vi "updateTestParameters.vi"(8 "error in (no error)":errorcluster, 11 "Model in":refnum<class "Model.lvclass">) -> (0 "error out":errorcluster, 3 "Model out":refnum<class "Model.lvclass">)   [LabVIEW 2015]
uses:
  ApplicationElements/TestMonitor/TestMonitor.lvclass
  Configuration/CycleProfileConfig.ctl
  Configuration/TestParameters.ctl
  ConfigurationThisComponent/ConfigurationThisComponent.lvclass
  Model.lvclass
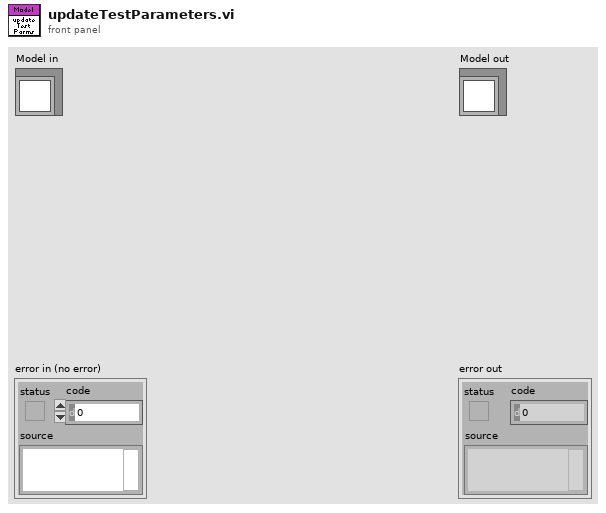
[diagram p1: front panel]
types:
  T1 = typedef "TestParameters.ctl" = cluster{"Number of cycles for complete test":u32, "Cycle profile":T2}
  T2 = typedef "CycleProfileConfig.ctl" = cluster{"Force Setpoint":dbl[unit][], "Pause After":dbl[unit][]}
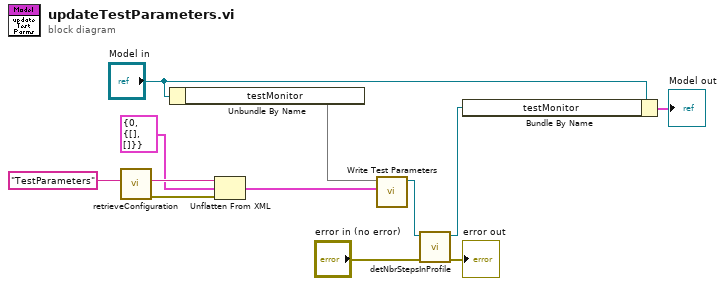
[diagram p0: block diagram]
diagram:
  n1 = call "retrieveConfiguration.vi"("configName"="TestParameters") -> ("error out"=w4:errorcluster, "xmlConfig"=w3:string)  [unwired: 8 in, 1 out]
  n2 = Unbundle By Name("Model in") -> ("testMonitor"=w11)
  n3 = Unflatten From XML(xml string=w3, type=T1 {"Number of cycles for complete test"=0, "Cycle profile"={"Force Setpoint"=[], "Pause After"=[]}} ("Test Parameters"), error in (no error)=w4) -> (value=w1:T1)  [unwired: 1 out]
  n4 = call "Write Test Parameters.vi"("Test Parameters"=w1, "TestMonitor in"=w11) -> ("TestMonitor out"=w10:refnum<class "TestMonitor.lvclass">)  [unwired: 9 in]
  n5 = call "detNbrStepsInProfile.vi"("error in (no error)"="error in (no error)", "TestMonitor in"=w10) -> ("error out"=→"error out":errorcluster, "TestMonitor out"=w9:refnum<class "TestMonitor.lvclass">)  [unwired: 8 in]
  n6 = Bundle By Name(cluster="Model in", "testMonitor"=w9) -> (→"Model out":cluster{})
